vi "Measurements Scan.vi"(8 "error in (no error)":errorcluster, 11 "Controller in":refnum<class "Controller.lvclass">) -> (0 "error out":errorcluster, 3 "Controller out":refnum<class "Controller.lvclass">)   [LabVIEW 2017, in "Controller Actor.lvlib" / "Controller.lvclass"]
uses:
  Controller.lvclass
  Controller.lvclass/Controller.ctl
  Accessors/Read Root Path.vi
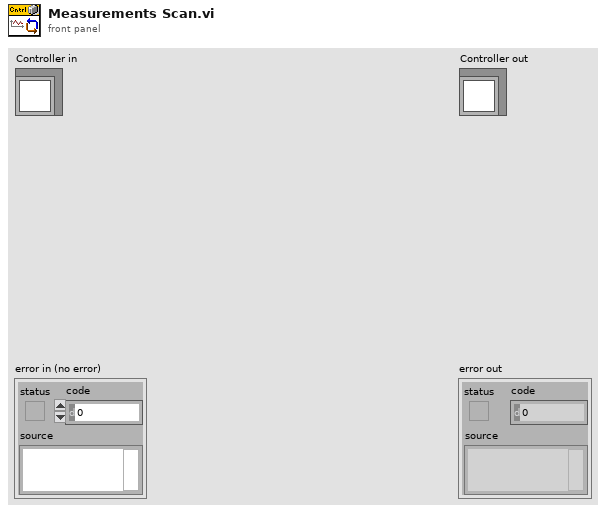
[diagram p1: front panel]
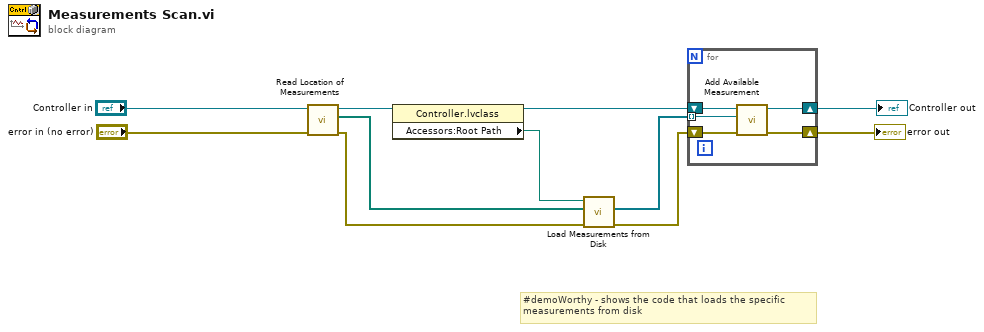
[diagram p0: block diagram]
diagram:
  # "#demoWorthy - shows the code that loads the specific\nmeasurements from disk"
  n1 = call "Read Location of Measurements.vi"("error in (no error)"="error in (no error)", "Controller in"="Controller in") -> ("error out"=w9:errorcluster, "Array of Measurement Location"=w8:path[], "Controller out"=w5:refnum<class "Controller.lvclass">)  [unwired: 7 in]
  n2 = property class="Controller.lvclass"(reference=w5) -> (reference out=w3:refnum<class "Controller.lvclass">, "Accessors:Root Path"=w4:path)  [unwired: 1 in, 1 out]
  n3 = call "Load Measurements from Disk.vi"("error in (no error)"=w9, "Array of paths (folders to scan or explicit files)"=w8, "base path"=w4) -> ("error out"=w6:errorcluster, "Available Measurements"=w7:refnum<class "Measurement.lvclass">[])  [unwired: 7 in]
  n4 = for {
    tunnel: w7 -> [w14] mode=indexing
    shift-right: [w15] -> w10
    shift-left: w3 -> [w16]
    shift-right: [w12] -> w11
    shift-left: w6 -> [w13]
    n5 = call "Add Available Measurement.vi"("error in (no error)"=w13, "Measurement.lvclass"=w14, "Controller in"=w16) -> ("error out"=w12:errorcluster, "Controller out"=w15:refnum<class "Controller.lvclass">)  [unwired: 7 in]
  }
  "error out" <- w11
  "Controller out" <- w10
